vi "CompileDUTPort.vi"(8 "error in (no error)":errorcluster, 11 "Device Item Ref in":T1 format="%.0x") -> (0 "error out":errorcluster, 2 "HW Info DUT Port":cluster{"CAN Port":string, "Baudrate":u64}, 3 "Device Item Ref out":T1 format="%.0x")   [LabVIEW 2018, in "CAN Gateway System Explorer.lvlib"]
uses:
  CAN Gateway System Explorer.lvlib
  <vilib>/NI Veristand/Custom Device API/Custom Device Item Ref.ctl
  Types/BR Cluster.ctl
  Shared/Constants.vi
  <vilib>/NI Veristand/Custom Device API/Get Item Property (String).vi
  <vilib>/NI Veristand/Custom Device API/Get Item Property (Variant).vi
  Shared/CAN Gateway Shared.lvlib
  <vilib>/NI Veristand/Custom Device API/Custom Device API.lvlib
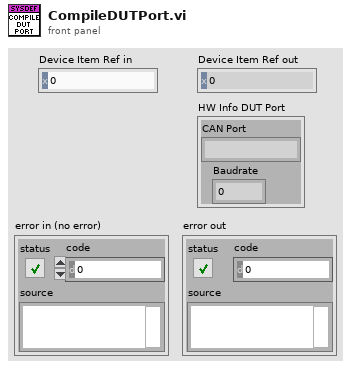
[diagram p1: front panel]
types:
  T1 = typedef "Custom Device API.lvlib/Custom Device Item Ref.ctl" = u64
  T2 = typedef "CAN Gateway System Explorer.lvlib/BR Cluster.ctl" = cluster{"BR Network-Port":u16, "BR Port Network":u16}
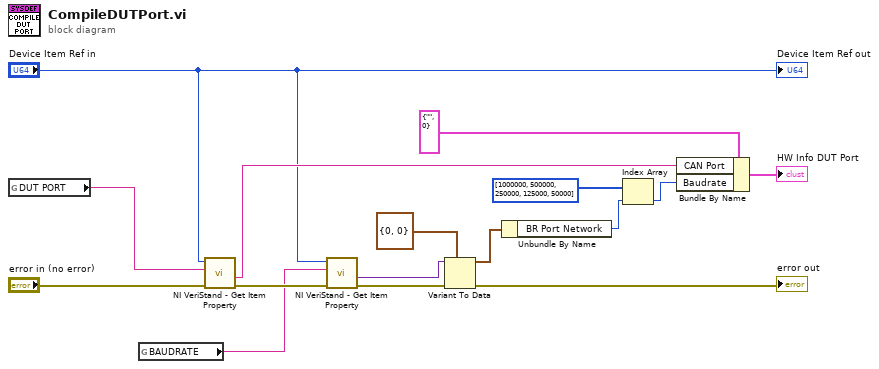
[diagram p0: block diagram]
diagram:
  n1 = global read "Constants.vi" "DUT PORT"() -> (w13:string)
  n2 = global read "Constants.vi" "BAUDRATE"() -> (w10:string)
  n3 = call-poly <vilib>:"NI VeriStand - Get Item Property.vi"("error in (no error)"="error in (no error)", "Property Name"=w13, "Item Ref in"="Device Item Ref in") -> ("error out"=w11:errorcluster, "Value"=w12:string)  [unwired: 5 in, 2 out]
  n4 = call-poly <vilib>:"NI VeriStand - Get Item Property.vi"("error in (no error)"=w11, "Property Name"=w10, "Item Ref in"="Device Item Ref in") -> ("error out"=w6:errorcluster, "Value"=w4:variant)  [unwired: 5 in, 2 out]
  n5 = Variant To Data(error in=w6, type=T2 {"BR Network-Port"=0, "BR Port Network"=0} ("BR Cluster"), Variant=w4) -> (data=w8:T2, error out=→"error out":errorcluster)
  n6 = Unbundle By Name(w8) -> ("BR Port Network"=w2:u16)
  n7 = Index Array(array=u64[] [1000000, 500000, 250000, 125000, 50000], index=w2) -> (element=w1:u64)
  n8 = Bundle By Name(cluster=cluster{"CAN Port":string, "Baudrate":u64} {"CAN Port"="", "Baudrate"=0} ("HW Info"), "CAN Port"=w12, "Baudrate"=w1) -> (→"HW Info DUT Port":cluster{"CAN Port":string, "Baudrate":u64})
  "Device Item Ref out" <- "Device Item Ref in"
